vi "logInternalCommand.vi"(8 "error in (no error)":errorcluster, 11 "SALCommunicator in":refnum<class "SALCommunicatorDL.lvclass">) -> (0 "error out":errorcluster, 3 "SALCommunicator out":refnum<class "SALCommunicatorDL.lvclass">)   [LabVIEW 2016, in "SALCommunicatorDL.lvclass"]
uses:
  SALCommunicatorDL.lvclass
  SALCommunicatorDL.lvclass/SALCommunicatorDL.ctl
  CommandConstruction/CommandConstruction.lvclass/CommandConstruction.ctl
  ts_sallv_exa/SALLV_EXA.lvlib
  CommandConstruction/CommandConstruction.lvclass
  SALCommand/SALCommand.lvclass
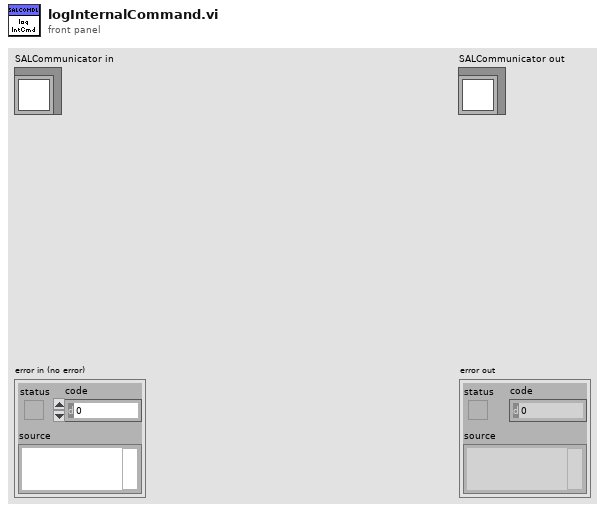
[diagram p1: front panel]
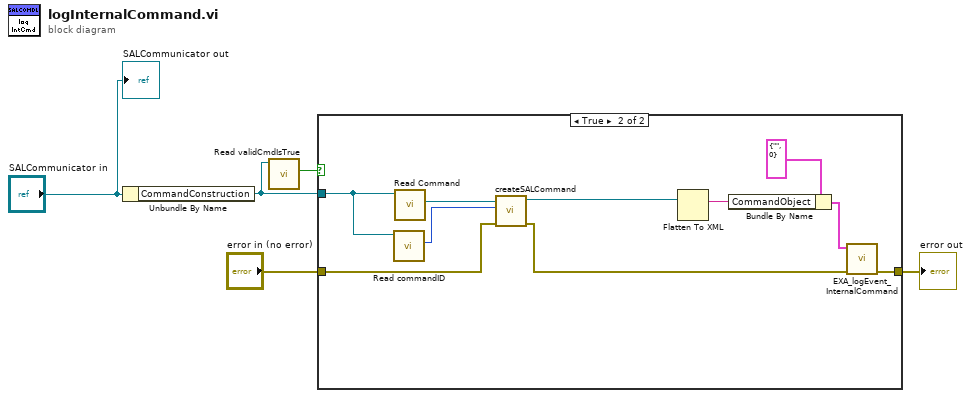
[diagram p0: block diagram]
diagram:
  n1 = Unbundle By Name("SALCommunicator in") -> ("CommandConstruction"=w1:refnum<class "CommandConstruction.lvclass">)
  n2 = call "Read validCmdIsTrue.vi"("CommandConstruction in"=w1) -> ("validCmdIsTrue"=w2:bool)  [unwired: 9 in, 1 out]
  n3 = case shown="True" w2 {
    tunnel: "error in (no error)" -> [w6 w11]
    tunnel: [w6 w16] -> w4
    tunnel: w1 -> [_ w13]
    frame False {
    }
    frame True {
      n4 = call "Read commandID.vi"("CommandConstruction in"=w13) -> ("commandID"=w9:i32)  [unwired: 9 in, 1 out]
      n5 = call "Read Command.vi"("CommandConstruction in"=w13) -> ("Command.lvclass"=w8:refnum<class "Command.lvclass">)  [unwired: 9 in, 1 out]
      n6 = call "createSALCommand.vi"("error in"=w11, "CommandID"=w9, "Command.lvclass"=w8) -> ("error out"=w10:errorcluster, "SALCommand.lvclass out"=w7:refnum<class "SALCommand.lvclass">)  [unwired: 7 in]
      n7 = Flatten To XML(anything=w7) -> (xml string=w14:string)
      n8 = Bundle By Name(cluster=cluster{"CommandObject":string, "priority":i32} {"CommandObject"="", "priority"=0}, "CommandObject"=w14) -> (w15:cluster{"CommandObject":string, "priority":i32})
      n9 = call "EXA_logEvent_InternalCommand.vi"("error in (no error)"=w10, "logevent_InternalCommand_Ctl"=w15) -> ("error out"=w16:errorcluster)  [unwired: 7 in, 2 out]
    }
  }
  "error out" <- w4
  "SALCommunicator out" <- "SALCommunicator in"
